vi "SysParamSetRef.vi"(4 "Init":bool, 5 "System Up Time in":refnum<vi>, 6 "Unit Add in":refnum<vi>, 7 "Op Amp Gain in":refnum<vi>, 8 "R Sense [ohms] in":refnum<vi>) -> (0 "Unit Add out":refnum<vi>, 1 "System Up Time out":refnum<vi>, 2 "Op Amp Gain out":refnum<vi>, 3 "R Sense [ohms] out":refnum<vi>)   [LabVIEW 2010]
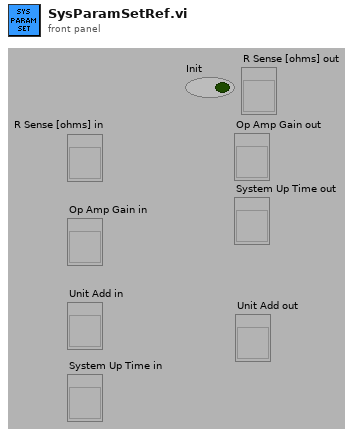
[diagram p1: front panel]
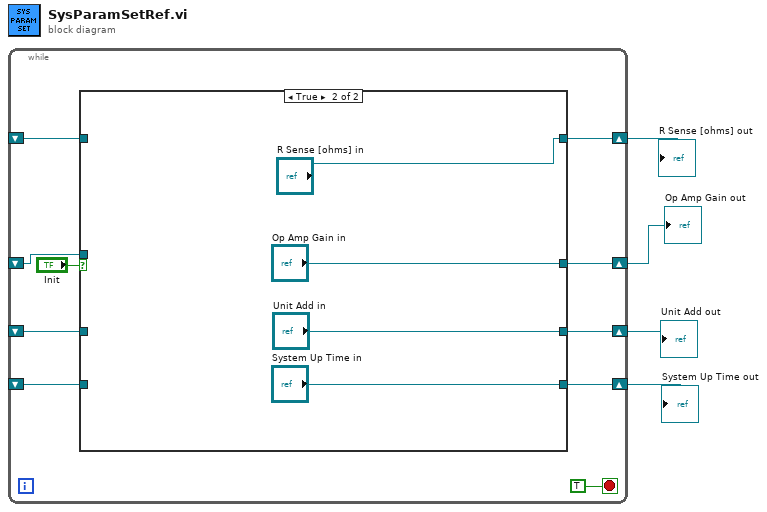
[diagram p0: block diagram]
diagram:
  n1 = while {
    shift-right: [w13] -> w1
    shift-left: _ -> [w9]
    shift-right: [w12] -> w4
    shift-left: _ -> [w8]
    shift-right: [w11] -> w3
    shift-left: _ -> [w7]
    shift-right: [w10] -> w2
    shift-left: _ -> [w6]
    stop <- TRUE stop-if-true
    n2 = case shown="True" "Init" {
      tunnel: [w18 "R Sense [ohms] in"] -> w13
      tunnel: [w17 "Op Amp Gain in"] -> w12
      tunnel: [w16 "Unit Add in"] -> w11
      tunnel: [w15 "System Up Time in"] -> w10
      tunnel: w9 -> [w18 _]
      tunnel: w8 -> [w17 _]
      tunnel: w7 -> [w16 _]
      tunnel: w6 -> [w15 _]
      frame False {
      }
      frame True {
      }
    }
  }
  "R Sense [ohms] out" <- w1
  "Op Amp Gain out" <- w4
  "Unit Add out" <- w3
  "System Up Time out" <- w2
